vi "Write URI.vi"(8 "error in (no error)":errorcluster, 10 "URI":string, 11 "Attribute.Config in":refnum<class "Attribute.Config.lvclass">) -> (0 "error out":errorcluster, 3 "Attribute.Config out":refnum<class "Attribute.Config.lvclass">)   [LabVIEW 2013, in "Attribute.Config.lvclass"]
uses:
  Attribute.Config.lvclass
  Attribute.Config.lvclass/Attribute.Config.ctl
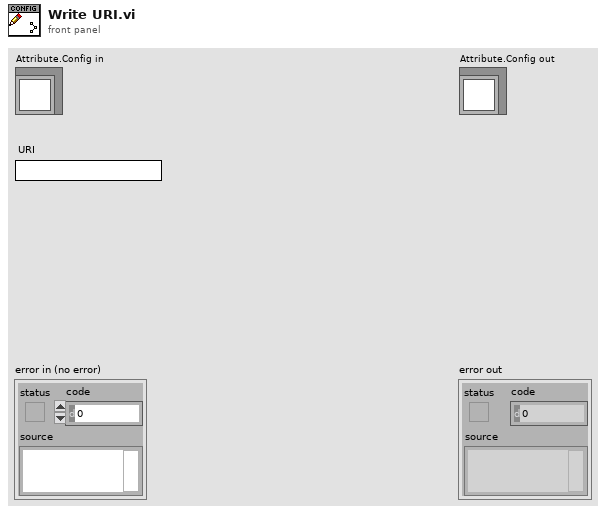
[diagram p1: front panel]
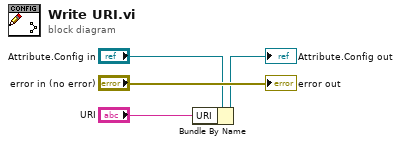
[diagram p0: block diagram]
diagram:
  n1 = Bundle By Name(cluster="Attribute.Config in", "URI"="URI") -> (→"Attribute.Config out":refnum<class "Attribute.Config.lvclass">)
  "error out" <- "error in (no error)"
